vi "Creat file by staion.vi"(6 "Header":string[](array[string]), 7 "basis as":enum16{"年_", "年_月_日_"}(ring), 11 "station":string) -> (3 "new file path (Not A Path if cancelled)":path caption="新建文件路径（取消时为非法路径）")   [LabVIEW 2014]
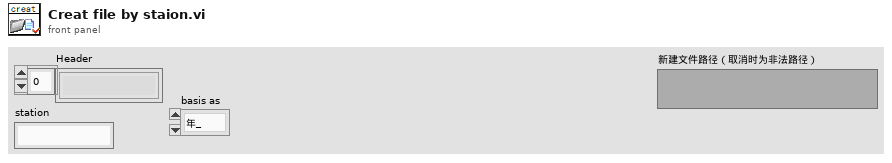
[diagram p1: front panel]
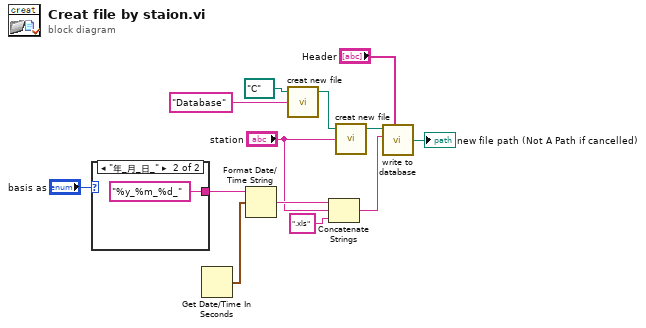
[diagram p0: block diagram]
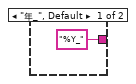
[diagram p2: hidden frame]
diagram:
  n1 = case shown="\"年_月_日_\"" "basis as" {
    tunnel: ["%Y_" ("时间格式字符串(%c)") "%y_%m_%d_" ("时间格式字符串(%c)")] -> w1
    frame "年_", Default {
    }
    frame "年_月_日_" {
    }
  }
  n2 = Get Date/Time In Seconds() -> (seconds since 1Jan1904=w9:timestamp)
  n3 = Format Date/Time String(time format string (%c)=w1, seconds (now)=w9) -> (date/time string=w8:string)  [unwired: 1 in]
  n4 = call "creat new file.vi"("file name"="Database", "path"=path "C:/") -> ("created path"=w11:path)  [unwired: 1 in, 2 out]
  n5 = Concatenate Strings(w8, "station", ".xls" ("字符串")) -> (w7:string)
  n6 = call "creat new file.vi"("file name"="station", "path"=w11) -> ("created path"=w10:path)  [unwired: 1 in, 2 out]
  n7 = call "write to database.vi"("Header"="Header", "file name"=w7, "path"=w10) -> ("new file path (Not A Path if cancelled)"=→"new file path (Not A Path if cancelled)":path)  [unwired: 3 in]
